vi "MCP4725.vi"() -> ()   [LabVIEW 2014]
uses:
  <vilib>/MakerHub/LINX/Private/Local IO/LinxI2cWrite.vi
  <vilib>/MakerHub/LINX/Public/Utilities/Check Channel.vi
  <vilib>/MakerHub/LINX/Public/Utilities/Open Serial.vi
  <vilib>/MakerHub/LINX/Private/Utilties/Generate Error.vi
  <vilib>/MakerHub/LINX/LMH-LINX.lvlib
panel:
  out "Gauge":dbl(knob) scale=0.0..5.0
  out "DAC Output":u16
  out "Device Name":string
  out "Error Out":errorcluster
  in  "millisecond multiple":u32
  in  "stop":bool
  in  "DAC Output Voltage":sgl min=0 max=5 step=0.001
  in  "Serial Port":refnum<visa-resource-name>="N/A"
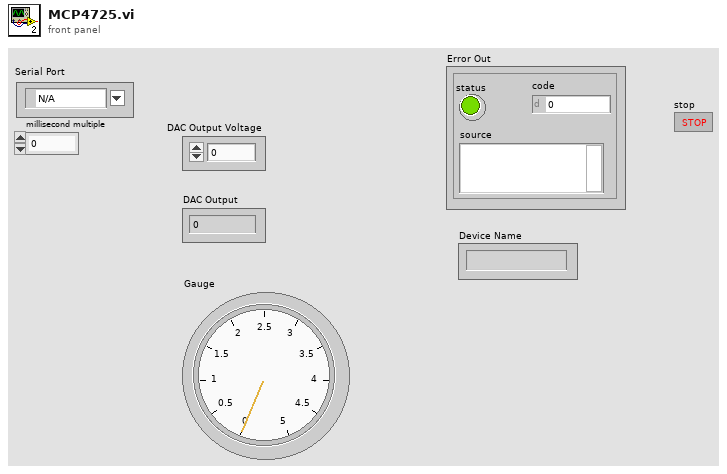
[diagram p1: front panel]
types:
  T1 = typedef "LMH-LINX.lvlib/LINX Ref.ctl" = cluster{"IO":T2, "Interface":T3, "LINX Device Config":T4}
  T2 = typedef "LMH-LINX.lvlib/Platform.ctl" = enum16{"Remote", "Local"}
  T3 = typedef "LMH-LINX.lvlib/Interface.ctl" = enum16{"Serial", "TCP"}
  T4 = typedef "LMH-LINX.lvlib/Device.lvlib/LINX Device Config.ctl" = cluster{"Interface":T3, "COM Port":refnum<visa-resource-name>, "TCP Configuration":T5, "Device Family":u8, "Device ID":u8, "Device Name":string, "TCP Ref":refnum<k5>, "Channels":T6}
  T5 = typedef "LMH-LINX.lvlib/Device.lvlib/TCP Config.ctl" = cluster{"IP Address":string, "Port":u16}
  T6 = typedef "LMH-LINX.lvlib/Channels.ctl" = cluster{"DI":u8[], "DO":u8[], "AI":u8[], "AO":u8[], "PWM":u8[], "QE":u8[], "UART":u8[], "I2C 2":u8[], "SPI":u8[], "CAN":u8[], "Servo":u8[], "AI Ref (V)":dbl, "AI Resolution (Bits)":u8, "AO Ref (V)":dbl, "AO Resolution (Bits)":u8}
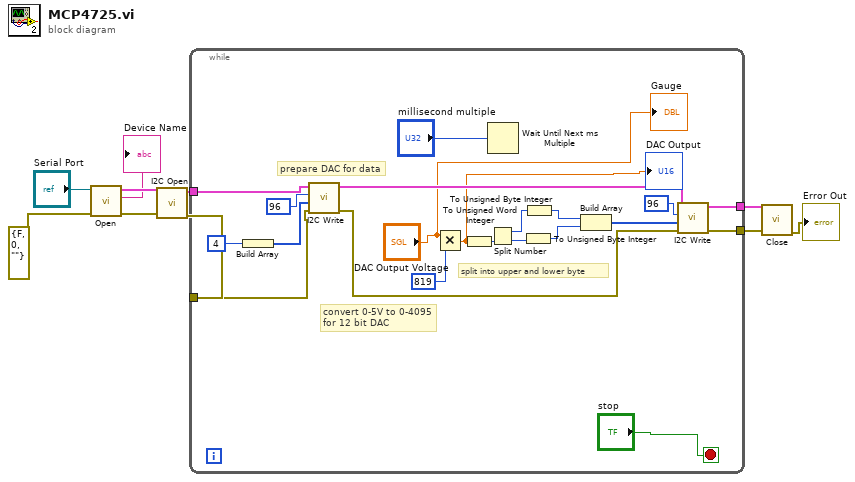
[diagram p0: block diagram]
diagram:
  n1 = call-poly <vilib>:"Open.vi"("Error In"=errorcluster {"status"=FALSE, "code"=0, "source"=""}, "Serial Port"="Serial Port") -> ("Error Out"=w8:errorcluster, "Device Name"=→"Device Name":string, "LINX Resource"=w9:T1)  [unwired: 7 in]
  n2 = call <vilib>:"I2C Open.vi"("Error In"=w8, "LINX Resource"=w9) -> ("Error Out"=w5:errorcluster, "LINX Resource"=w6:T1)  [unwired: 8 in]
  n3 = while {
    tunnel: w6 -> [w29]
    tunnel: w5 -> [w28]
    tunnel: [w31] -> w2
    tunnel: [w30] -> w1
    stop <- "stop" stop-if-true
    # "prepare DAC for data"
    # "convert 0-5V to 0-4095\nfor 12 bit DAC"
    # "split into upper and lower byte"
    n4 = Build Array(u8 4) -> (w12:u8[])
    n5 = call <vilib>:"I2C Write.vi"("Error In"=w28, "Data"=w12, "I2C Slave Address (0)"=u8 96, "LINX Resource"=w29) -> ("Error Out"=w16:errorcluster, "LINX Resource"=w15:T1)  [unwired: 6 in]
    n6 = Multiply(x="DAC Output Voltage", y=u32 819) -> (x*y=w14:sgl)
    "DAC Output" <- w14
    n7 = To Unsigned Word Integer(number=w14) -> (unsigned 16bit integer=w19:u16)
    n8 = Wait Until Next ms Multiple(millisecond multiple="millisecond multiple") -> ()  [unwired: 1 out]
    n9 = Split Number(x=w19) -> (hi(x)=w20:u8, lo(x)=w25:u8)
    n10 = To Unsigned Byte Integer(number=w25) -> (unsigned 8bit integer=w22:u8)
    n11 = To Unsigned Byte Integer(number=w20) -> (unsigned 8bit integer=w23:u8)
    n12 = Build Array(w23, w22) -> (w21:u8[])
    n13 = call <vilib>:"I2C Write.vi"("Error In"=w16, "Data"=w21, "I2C Slave Address (0)"=u8 96, "LINX Resource"=w15) -> ("Error Out"=w30:errorcluster, "LINX Resource"=w31:T1)  [unwired: 6 in]
    "Gauge" <- "DAC Output Voltage"
  }
  n14 = call <vilib>:"Close.vi"("Error In"=w1, "LINX Resource"=w2) -> ("Error Out"=→"Error Out":errorcluster)  [unwired: 9 in]
